vi "Decoder Display.vi"(8 "error IO":errorcluster, 11 "all rows":string[][](array[string])) -> (0 "error IO 2":errorcluster, 3 "array":string[][](array[string]))   [LabVIEW 2022 SP3]
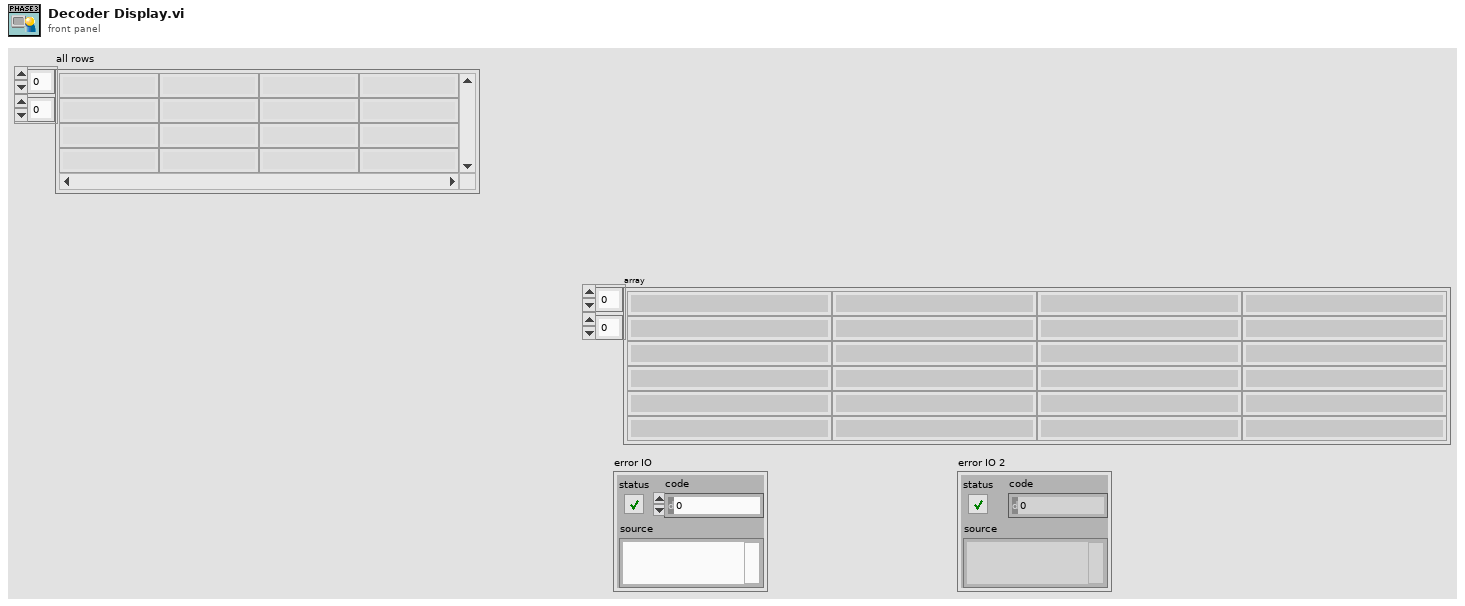
[diagram p1: front panel]
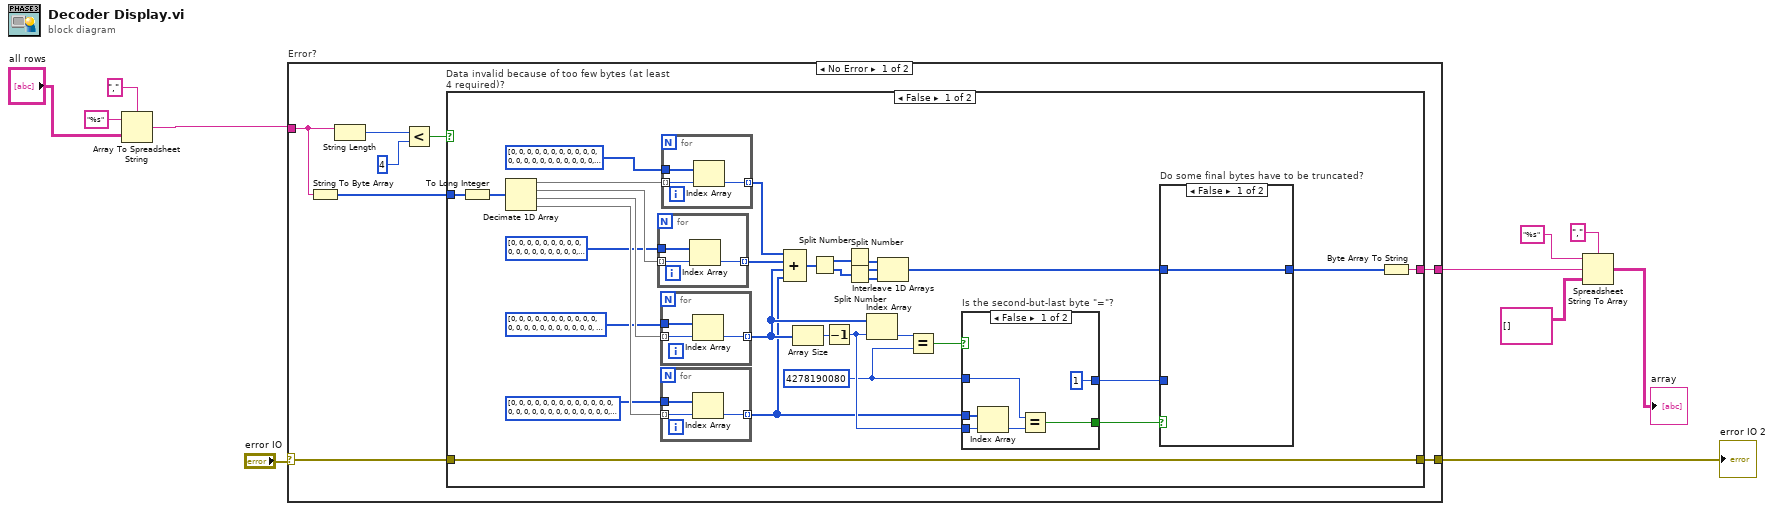
[diagram p0: block diagram]
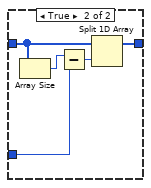
[diagram p2: hidden frame]
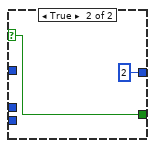
[diagram p3: hidden frame]
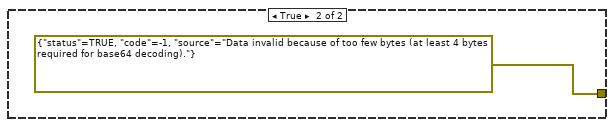
[diagram p4: hidden frame]
diagram:
  n1 = Array To Spreadsheet String(delimiter (Tab)=",", array="all rows", 3:"%s" ("format string")) -> (spreadsheet string=w5:string)
  n2 = case "Error?" shown="No Error" "error IO" {
    selector: "error IO" -> [w14 w78]
    tunnel: w5 -> [w18 _]
    tunnel: [w13 w78] -> w4
    tunnel: [w12 _] -> w2
    frame No Error {
      n3 = String To Byte Array(string=w18) -> (unsigned byte array=w17:u8[])
      n4 = String Length(string=w18) -> (length=w15:i32)
      n5 = Less?(x=w15, y=4) -> (x < y?=w16:bool)
      n6 = case "Data invalid because of too few bytes (at least 4 required)?" shown="False" w16 {
        tunnel: w17 -> [w32 _]
        tunnel: [w50 _] -> w12
        tunnel: [w20 errorcluster {"status"=TRUE, "code"=-1, "source"="Data invalid because of too few bytes (at least 4 bytes required for base64 decoding)."} ("error IO")] -> w13
        tunnel: w14 -> [w20 _]
        frame False {
          w25 = u32 4278190080 ("y")
          n7 = To Long Integer(number=w32) -> (32bit integer=w49:i32[])
          n8 = Decimate 1D Array(w49) -> (w38:i32[], w48:i32[], w39:i32[], w37:i32[])
          n9 = for {
            tunnel: w48 -> [w72] mode=indexing
            tunnel: u32[] [0, 0, 0, 0, 0, 0, 0, 0, 0, 0, 0, 0, 0, 0, 0, 0, 0, 0, 0, 0, 0, 0, 0, 0, 0, 0, 0, 0, 0, 0, 0, 0, 0, 0, 0, 0, 0, 0, 0, 0, 0, 0, 0, 253952, 0, 0, 0, 258048, 212992, 217088, 221184, 225280, 229376, 233472, 237568, 241664, 245760, 249856, 0, 0, 0, 0, 0, 0, 0, 0, 4096, 8192, 12288, 16384, 20480, 24576, 28672, 32768, 36864, 40960, 45056, 49152, 53248, 57344, 61440, 65536, 69632, 73728, 77824, 81920, 86016, 90112, 94208, 98304, 102400, 0, 0, 0, 0, 0, 0, 106496, 110592, 114688, 118784, 122880, 126976, 131072, 135168, 139264, 143360, 147456, 151552, 155648, 159744, 163840, 167936, 172032, 176128, 180224, 184320, 188416, 192512, 196608, 200704, 204800, 208896, 0, 0, 0, 0, 0, 0, 0, 0, 0, 0, 0, 0, 0, 0, 0, 0, 0, 0, 0, 0, 0, 0, 0, 0, 0, 0, 0, 0, 0, 0, 0, 0, 0, 0, 0, 0, 0, 0, 0, 0, 0, 0, 0, 0, 0, 0, 0, 0, 0, 0, 0, 0, 0, 0, 0, 0, 0, 0, 0, 0, 0, 0, 0, 0, 0, 0, 0, 0, 0, 0, 0, 0, 0, 0, 0, 0, 0, 0, 0, 0, 0, 0, 0, 0, 0, 0, 0, 0, 0, 0, 0, 0, 0, 0, 0, 0, 0, 0, 0, 0, 0, 0, 0, 0, 0, 0, 0, 0, 0, 0, 0, 0, 0, 0, 0, 0, 0, 0, 0, 0, 0, 0, 0, 0, 0, 0, 0, 0, 0, 0, 0, 0, 0] ("array 3") -> [w73]
            tunnel: [w71] -> w46 mode=indexing
            n10 = Index Array(array=w73, index=w72) -> (element=w71:u32)
          }
          n11 = for {
            tunnel: u32[] [0, 0, 0, 0, 0, 0, 0, 0, 0, 0, 0, 0, 0, 0, 0, 0, 0, 0, 0, 0, 0, 0, 0, 0, 0, 0, 0, 0, 0, 0, 0, 0, 0, 0, 0, 0, 0, 0, 0, 0, 0, 0, 0, 3968, 0, 0, 0, 4032, 3328, 3392, 3456, 3520, 3584, 3648, 3712, 3776, 3840, 3904, 0, 0, 0, 4278190080, 0, 0, 0, 0, 64, 128, 192, 256, 320, 384, 448, 512, 576, 640, 704, 768, 832, 896, 960, 1024, 1088, 1152, 1216, 1280, 1344, 1408, 1472, 1536, 1600, 0, 0, 0, 0, 0, 0, 1664, 1728, 1792, 1856, 1920, 1984, 2048, 2112, 2176, 2240, 2304, 2368, 2432, 2496, 2560, 2624, 2688, 2752, 2816, 2880, 2944, 3008, 3072, 3136, 3200, 3264, 0, 0, 0, 0, 0, 0, 0, 0, 0, 0, 0, 0, 0, 0, 0, 0, 0, 0, 0, 0, 0, 0, 0, 0, 0, 0, 0, 0, 0, 0, 0, 0, 0, 0, 0, 0, 0, 0, 0, 0, 0, 0, 0, 0, 0, 0, 0, 0, 0, 0, 0, 0, 0, 0, 0, 0, 0, 0, 0, 0, 0, 0, 0, 0, 0, 0, 0, 0, 0, 0, 0, 0, 0, 0, 0, 0, 0, 0, 0, 0, 0, 0, 0, 0, 0, 0, 0, 0, 0, 0, 0, 0, 0, 0, 0, 0, 0, 0, 0, 0, 0, 0, 0, 0, 0, 0, 0, 0, 0, 0, 0, 0, 0, 0, 0, 0, 0, 0, 0, 0, 0, 0, 0, 0, 0, 0, 0, 0, 0, 0, 0, 0, 0] ("array 2") -> [w70]
            tunnel: [w69] -> w30 mode=indexing
            tunnel: w39 -> [w68] mode=indexing
            n12 = Index Array(array=w70, index=w68) -> (element=w69:u32)
          }
          n13 = for {
            tunnel: u32[] [0, 0, 0, 0, 0, 0, 0, 0, 0, 0, 0, 0, 0, 0, 0, 0, 0, 0, 0, 0, 0, 0, 0, 0, 0, 0, 0, 0, 0, 0, 0, 0, 0, 0, 0, 0, 0, 0, 0, 0, 0, 0, 0, 62, 0, 0, 0, 63, 52, 53, 54, 55, 56, 57, 58, 59, 60, 61, 0, 0, 0, 4278190080, 0, 0, 0, 0, 1, 2, 3, 4, 5, 6, 7, 8, 9, 10, 11, 12, 13, 14, 15, 16, 17, 18, 19, 20, 21, 22, 23, 24, 25, 0, 0, 0, 0, 0, 0, 26, 27, 28, 29, 30, 31, 32, 33, 34, 35, 36, 37, 38, 39, 40, 41, 42, 43, 44, 45, 46, 47, 48, 49, 50, 51, 0, 0, 0, 0, 0, 0, 0, 0, 0, 0, 0, 0, 0, 0, 0, 0, 0, 0, 0, 0, 0, 0, 0, 0, 0, 0, 0, 0, 0, 0, 0, 0, 0, 0, 0, 0, 0, 0, 0, 0, 0, 0, 0, 0, 0, 0, 0, 0, 0, 0, 0, 0, 0, 0, 0, 0, 0, 0, 0, 0, 0, 0, 0, 0, 0, 0, 0, 0, 0, 0, 0, 0, 0, 0, 0, 0, 0, 0, 0, 0, 0, 0, 0, 0, 0, 0, 0, 0, 0, 0, 0, 0, 0, 0, 0, 0, 0, 0, 0, 0, 0, 0, 0, 0, 0, 0, 0, 0, 0, 0, 0, 0, 0, 0, 0, 0, 0, 0, 0, 0, 0, 0, 0, 0, 0, 0, 0, 0, 0, 0, 0, 0, 0] ("Array") -> [w67]
            tunnel: [w66] -> w28 mode=indexing
            tunnel: w37 -> [w65] mode=indexing
            n14 = Index Array(array=w67, index=w65) -> (element=w66:u32)
          }
          n15 = for {
            tunnel: w38 -> [w75] mode=indexing
            tunnel: u32[] [0, 0, 0, 0, 0, 0, 0, 0, 0, 0, 0, 0, 0, 0, 0, 0, 0, 0, 0, 0, 0, 0, 0, 0, 0, 0, 0, 0, 0, 0, 0, 0, 0, 0, 0, 0, 0, 0, 0, 0, 0, 0, 0, 16252928, 0, 0, 0, 16515072, 13631488, 13893632, 14155776, 14417920, 14680064, 14942208, 15204352, 15466496, 15728640, 15990784, 0, 0, 0, 0, 0, 0, 0, 0, 262144, 524288, 786432, 1048576, 1310720, 1572864, 1835008, 2097152, 2359296, 2621440, 2883584, 3145728, 3407872, 3670016, 3932160, 4194304, 4456448, 4718592, 4980736, 5242880, 5505024, 5767168, 6029312, 6291456, 6553600, 0, 0, 0, 0, 0, 0, 6815744, 7077888, 7340032, 7602176, 7864320, 8126464, 8388608, 8650752, 8912896, 9175040, 9437184, 9699328, 9961472, 10223616, 10485760, 10747904, 11010048, 11272192, 11534336, 11796480, 12058624, 12320768, 12582912, 12845056, 13107200, 13369344, 0, 0, 0, 0, 0, 0, 0, 0, 0, 0, 0, 0, 0, 0, 0, 0, 0, 0, 0, 0, 0, 0, 0, 0, 0, 0, 0, 0, 0, 0, 0, 0, 0, 0, 0, 0, 0, 0, 0, 0, 0, 0, 0, 0, 0, 0, 0, 0, 0, 0, 0, 0, 0, 0, 0, 0, 0, 0, 0, 0, 0, 0, 0, 0, 0, 0, 0, 0, 0, 0, 0, 0, 0, 0, 0, 0, 0, 0, 0, 0, 0, 0, 0, 0, 0, 0, 0, 0, 0, 0, 0, 0, 0, 0, 0, 0, 0, 0, 0, 0, 0, 0, 0, 0, 0, 0, 0, 0, 0, 0, 0, 0, 0, 0, 0, 0, 0, 0, 0, 0, 0, 0, 0, 0, 0, 0, 0, 0, 0, 0, 0, 0, 0] ("array 4") -> [w76]
            tunnel: [w74] -> w47 mode=indexing
            n16 = Index Array(array=w76, index=w75) -> (element=w74:u32)
          }
          n17 = Compound Arithmetic op=ADD(w47, w46, w30, w28) -> (w44:u32[])
          n18 = Array Size(array=w30) -> (size(s)=w31:i32)
          n19 = Split Number(x=w44) -> (hi(x)=w45:u16[], lo(x)=w43:u16[])
          n20 = Decrement(x=w31) -> (x-1=w29:i32)
          n21 = Split Number(x=w45) -> (lo(x)=w40:u8[])  [unwired: 1 out]
          n22 = Split Number(x=w43) -> (hi(x)=w41:u8[], lo(x)=w42:u8[])
          n23 = Index Array(array=w30, index=w29) -> (element=w27:u32)
          n24 = Interleave 1D Arrays(w40, w41, w42) -> (w22:u8[])
          n25 = Equal?(x=w27, y=w25) -> (x = y?=w26:bool)
          n26 = case "Is the second-but-last byte \"=\"?" shown="False" w26 {
            selector: w26 -> [_ w63]
            tunnel: w29 -> [w62 _]
            tunnel: w28 -> [w61 _]
            tunnel: w25 -> [w59 _]
            tunnel: [w58 w63] -> w24
            tunnel: [1 2] -> w23
            frame False {
              n27 = Index Array(array=w61, index=w62) -> (element=w60:u32)
              n28 = Equal?(x=w59, y=w60) -> (x = y?=w58:bool)
            }
            frame True {
            }
          }
          n29 = case "Do some final bytes have to be truncated?" shown="False" w24 {
            tunnel: w23 -> [_ w56]
            tunnel: w22 -> [w51 w52]
            tunnel: [w51 w54] -> w21
            frame False {
            }
            frame True {
              n30 = Array Size(array=w52) -> (size(s)=w53:i32)
              n31 = Subtract(x=w53, y=w56) -> (x-y=w55:i32)
              n32 = Split 1D Array(array=w52, index=w55) -> (first subarray=w54:u8[])  [unwired: 1 out]
            }
          }
          n33 = Byte Array To String(unsigned byte array=w21) -> (string=w50:string)
        }
        frame True {
        }
      }
    }
    frame Error {
    }
  }
  "error IO 2" <- w4
  n34 = Spreadsheet String To Array(delimiter (Tab)=",", format string="%s", spreadsheet string=w2, array type (2D Dbl)=string[][] [] ("all rows")) -> (array=→"array":string[][])
